vi "WorkorderHandler_SaveFile.vi"(8 "error in (no error)":errorcluster, 11 "reference":T1) -> (0 "error out":errorcluster, 3 "duplicate reference":T1)   [LabVIEW 2011]
uses:
  DataStructures/WorkorderHandler_ObjectReference.ctl
  Strict Type Controls/Settings Operation.ctl
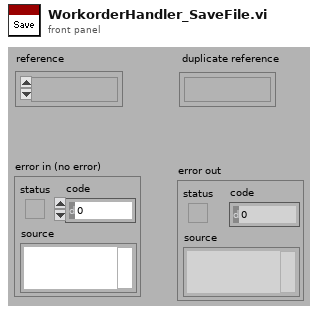
[diagram p1: front panel]
types:
  T1 = typedef "WorkorderHandler_ObjectReference.ctl" = refnum<k1>
  T2 = typedef "WorkorderHandler_ObjectData.ctl" = cluster{"Table":string[][], "Script":string, "Order":string, "No":string, "Time":dbl}
  T3 = typedef "Settings Operation.ctl" = enum8{"Get Value", "Set Value", "Read File", "Write File", "Write Stored Value"}
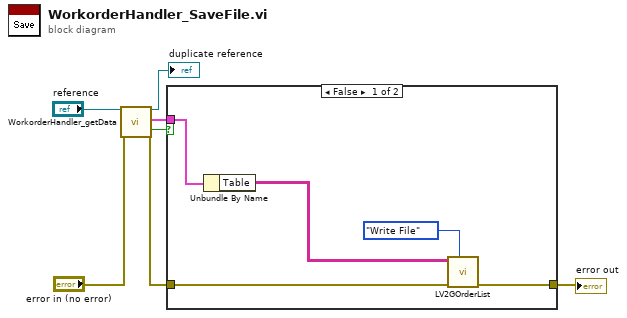
[diagram p0: block diagram]
diagram:
  n1 = call "WorkorderHandler_getData.vi"("reference"="reference", "error in (no error)"="error in (no error)") -> ("duplicate reference"=→"duplicate reference":T1, "data"=w5:T2, "timed out?"=w1:bool, "error out"=w2:errorcluster)  [unwired: 1 in, 13 out]
  n2 = case shown="False" w1 {
    tunnel: w5 -> [w12 _]
    tunnel: [w8 w13] -> w4
    tunnel: w2 -> [w9 w13]
    frame False {
      n3 = Unbundle By Name(w12) -> ("Table"=w10:string[][])
      n4 = call "LV2GOrderList.vi"("Operation"=Settings_Operation."Write File", "error in (no error)"=w9, "Orders"=w10) -> ("error out"=w8:errorcluster)  [unwired: 8 out]
    }
    frame True {
      # "Error or Timed Out"
    }
  }
  "error out" <- w4
